vi "OCR_Find Text Row Locations.vi"(8 "Error":errorcluster, 9 "Color Array":T1[](array[typedef]), 10 "Row Type Array":T3[](array[typedef]), 11 "Frame Color":u32(colorbox)) -> (0 "Error Out":errorcluster, 1 "All Good Out":bool, 2 "Body Cluster Out":T2, 3 "Color Array Out":T1[](array[typedef]), 4 "Header Out":bool)   [LabVIEW 2009]
doc: "Finds Text Row location of each text line in the icon"
uses:
  Controls/Enum/ENUM_Line Letter Type.ctl
  Controls/Cluster/Cluster_Line Location and status.ctl
  Controls/Cluster/Cluster_Text Color Set.ctl
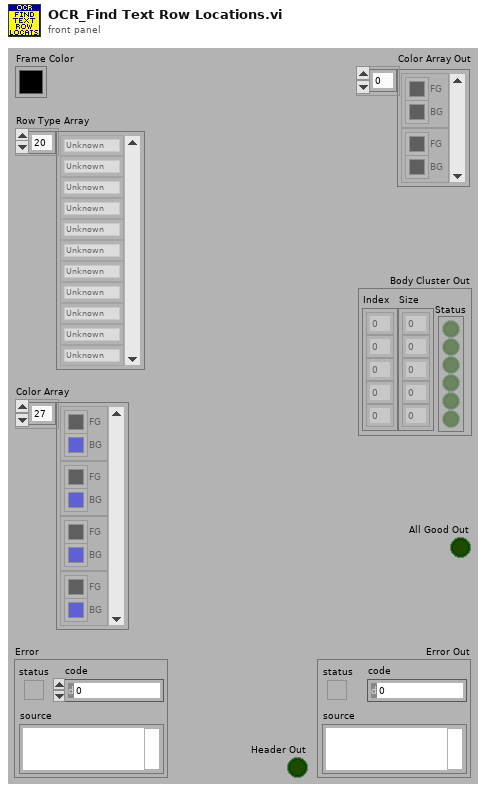
[diagram p1: front panel]
types:
  T1 = typedef "Cluster_Text Color Set.ctl" = cluster{"BG":u32, "FG":u32}
  T2 = typedef "Cluster_Line Location and status.ctl" = cluster{"Index":i16[], "Status":bool[], "Size":i32[]}
  T3 = typedef "ENUM_Line Letter Type.ctl" = enum16{"Unknown", "Letter", "Seperator", "Seperator or Letter"}
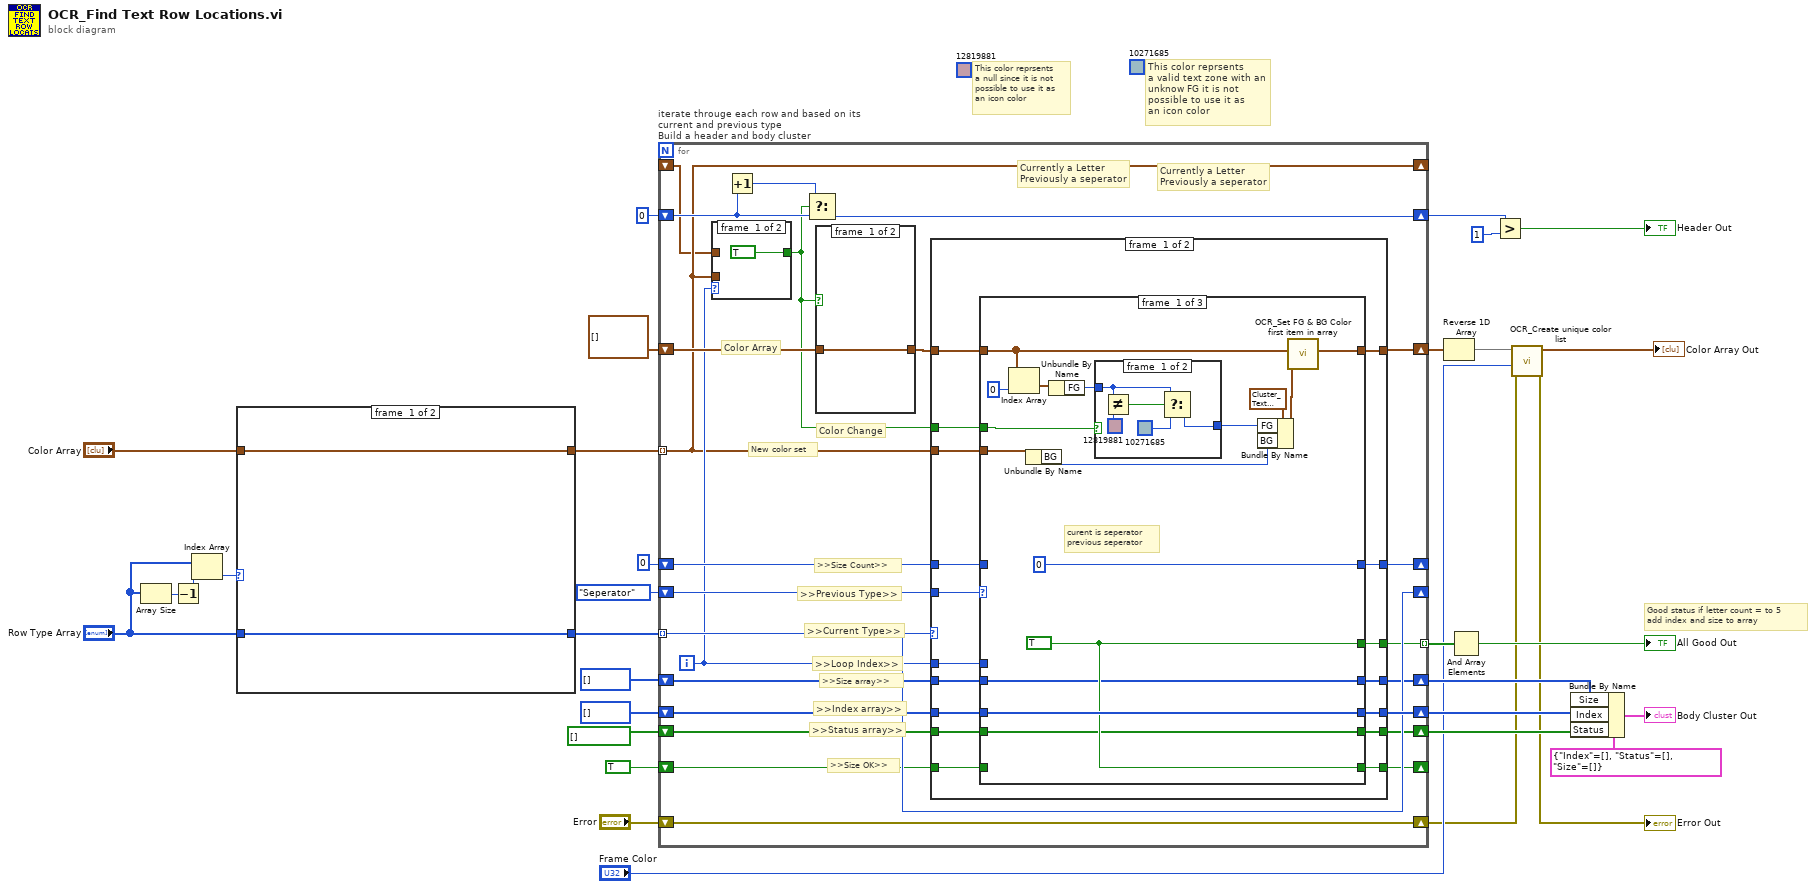
[diagram p0: block diagram]
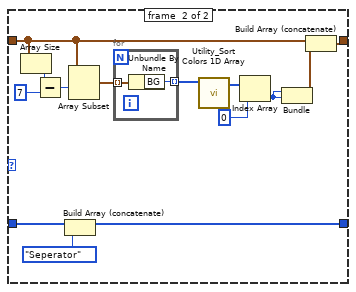
[diagram p2: hidden frame]
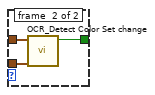
[diagram p3: hidden frame]
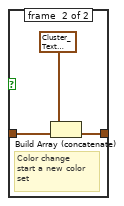
[diagram p4: hidden frame]
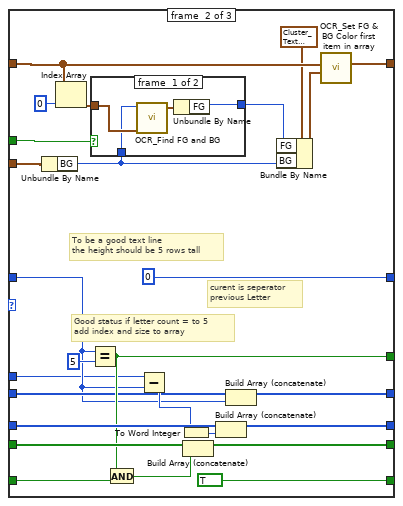
[diagram p6: hidden frame]
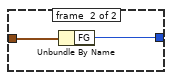
[diagram p7: hidden frame]
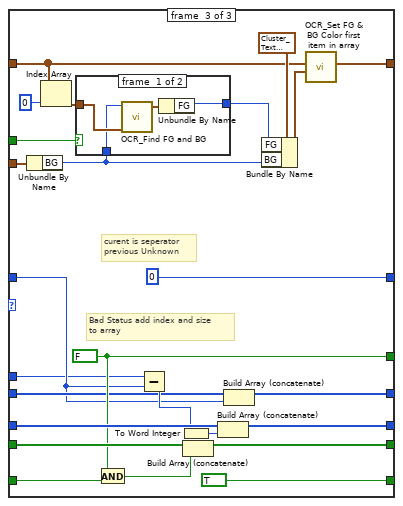
[diagram p8: hidden frame]
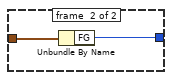
[diagram p9: hidden frame]
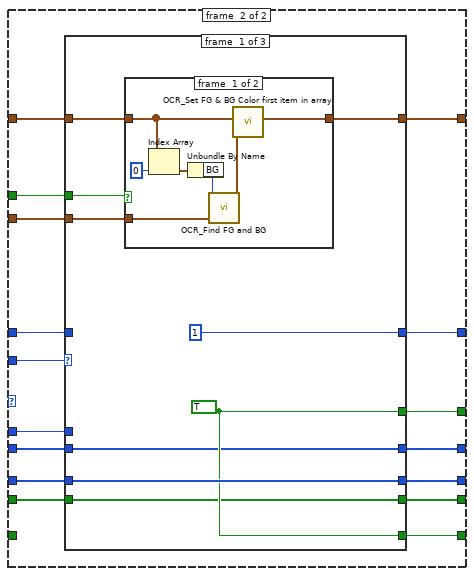
[diagram p10: hidden frame]
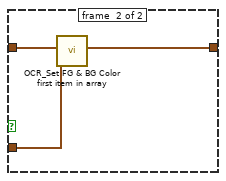
[diagram p11: hidden frame]
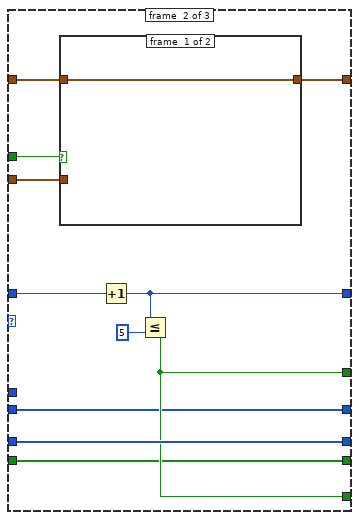
[diagram p12: hidden frame]
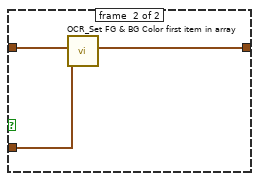
[diagram p13: hidden frame]
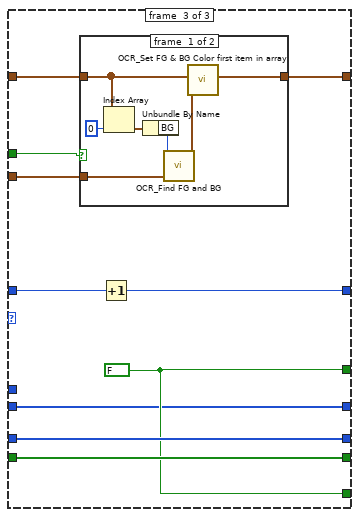
[diagram p14: hidden frame]
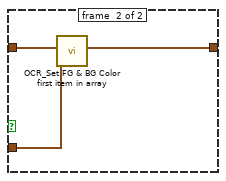
[diagram p15: hidden frame]
diagram:
  (unwired) u32 10271685 ("Unknown FG")
  (unwired) u32 12819881
  # "This color reprsents\na valid text zone with an \nunknow FG it is not\npossible to use it as\nan icon color"
  # "This color reprsents\na null since it is not\npossible to use it as\nan icon color"
  # "Good status if letter count = to 5\nadd index and size to array"
  n1 = Array Size(array="Row Type Array") -> (size(s)=w5:i32)
  n2 = Decrement(x=w5) -> (x-1=w4:i32)
  n3 = Index Array(array="Row Type Array", index=w4) -> (element=w1:T3)
  n4 = case shown="Default" w1 {
    tunnel: "Color Array" -> [w34 w44]
    tunnel: [w34 w48] -> w6
    tunnel: "Row Type Array" -> [w33 w47]
    tunnel: [w33 w46] -> w3
    frame #0 {
    }
    frame #1 {
      n5 = Array Size(array=w44) -> (size(s)=w43:i32)
      n6 = Subtract(x=w43, y=7) -> (x-y=w41:i32)
      n7 = Build Array (concatenate)(w47, ENUM_Line_Letter_Type."Seperator" ("element")) -> (w46:T3[])
      n8 = Array Subset(array=w44, index=w41) -> (w40:T1[])  [unwired: 1 in]
      n9 = for {
        tunnel: w40 -> [w50] mode=indexing
        tunnel: [w49] -> w39 mode=indexing
        n10 = Unbundle By Name(w50) -> ("BG"=w49:u32)
      }
      n11 = call "Utility_Sort Colors 1D Array.vi"("Colors"=w39) -> ("Sorted By Quantity Out"=w38:u32[])  [unwired: 8 in, 2 out]
      n12 = Index Array(array=w38, index=0) -> (element=w37:u32)
      n13 = Bundle(w37, w37) -> (w35:cluster{u32, u32})  [unwired: 1 in]
      n14 = Build Array (concatenate)(w44, w35) -> (w48:T1[])
    }
  }
  n15 = for "iterate througe each row and based on its current and previous type\nBuild a header and body cluster" {
    tunnel: w3 -> [w68] mode=indexing
    shift-right: [w74] -> w9
    shift-left: "Error" -> [w74]
    shift-right: [w71] -> _
    shift-left: 0 -> [w72]
    shift-right: [w69] -> w22
    shift-left: i16[] [] -> [w70]
    shift-right: [w68] -> _
    shift-left: ENUM_Line_Letter_Type."Seperator" ("Type Out") -> [w73]
    tunnel: [w67] -> w28 mode=indexing
    shift-right: [w65] -> w20
    shift-left: bool[] [] -> [w64]
    shift-right: [w63] -> _
    shift-left: TRUE -> [w66]
    shift-right: [w61] -> w21
    shift-left: i32[] [] -> [w62]
    tunnel: w6 -> [w52] mode=indexing
    shift-right: [w60] -> w17
    shift-left: T1[] [] -> [w55]
    shift-right: [w57] -> w15
    shift-left: 0 -> [w58]
    shift-right: [w52] -> _
    shift-left: _ -> [w51]
    i -> [w54]
    # ">>Loop Index>>"
    # "Currently a Letter\nPreviously a seperator"
    # "Currently a Letter\nPreviously a seperator"
    # "Color Change"
    # "New color set"
    # "Color Array"
    # ">>Size Count>>"
    # ">>Current Type>>"
    # ">>Previous Type>>"
    # ">>Size OK>>"
    # ">>Status array>>"
    # ">>Index array>>"
    # ">>Size array>>"
    n16 = case shown="1.." w54 {
      tunnel: [TRUE w77] -> w53
      tunnel: w52 -> [_ w78]
      tunnel: w51 -> [_ w76]
      frame #0 {
      }
      frame #1 {
        n17 = call "OCR_Detect Color Set change.vi"("New Color Set"=w78, "Previous Color Set"=w76) -> ("Color Change Out"=w77:bool)  [unwired: 9 in]
      }
    }
    n18 = Increment(x=w58) -> (x+1=w59:i32)
    n19 = Select(t=w59, s=w53, f=w58) -> (s? t:f=w57:i32)
    n20 = case shown="True" w53 {
      tunnel: w55 -> [w79 w82]
      tunnel: [w79 w81] -> w56
      frame #0 {
      }
      frame #1 {
        # "Color change\nstart a new color\nset"
        n21 = Build Array (concatenate)(T1 {"BG"=12819881, "FG"=12819881} ("Color Set"), w82) -> (w81:T1[])
      }
    }
    n22 = case shown="\"Seperator\", \"Seperator or Letter\"" w68 {
      tunnel: w73 -> [w95 w195]
      tunnel: w72 -> [w98 w199]
      tunnel: [w99 w200] -> w71
      tunnel: w54 -> [w87 w198]
      tunnel: w70 -> [w97 w197]
      tunnel: [w96 w196] -> w69
      tunnel: [w94 w194] -> w67
      tunnel: w66 -> [w93 _]
      tunnel: [w92 w192] -> w65
      tunnel: w64 -> [w91 w191]
      tunnel: [w90 w193] -> w63
      tunnel: w62 -> [w89 w190]
      tunnel: [w88 w189] -> w61
      tunnel: w56 -> [w85 w188]
      tunnel: [w83 w187] -> w60
      tunnel: w52 -> [w84 w185]
      tunnel: w53 -> [w86 w186]
      frame #0 {
        n23 = case shown="\"Letter\"" w95 {
          tunnel: [0 0 0] -> w99
          tunnel: w98 -> [_ w133 w165]
          tunnel: w87 -> [_ w132 w164]
          tunnel: w97 -> [w114 w145 w177]
          tunnel: [w114 w144 w176] -> w96
          tunnel: [w113 w137 w168] -> w94
          tunnel: w93 -> [_ w143 w175]
          tunnel: [w112 w142 w174] -> w92
          tunnel: w91 -> [w112 w141 w173]
          tunnel: [w113 TRUE TRUE] -> w90
          tunnel: [w111 w135 w166] -> w88
          tunnel: w89 -> [w111 w134 w167]
          tunnel: w86 -> [w108 w122 w156]
          tunnel: w85 -> [w105 w126 w159]
          tunnel: [w104 w125 w163] -> w83
          tunnel: w84 -> [w106 w123 w162]
          frame #0 {
            w113 = TRUE
            # "curent is seperator\nprevious seperator"
            n24 = Index Array(array=w105, index=0) -> (element=w109:T1)
            n25 = Unbundle By Name(w106) -> ("BG"=w100:u32)
            n26 = Unbundle By Name(w109) -> ("FG"=w107:u32)
            n27 = case shown="False" w108 {
              tunnel: w107 -> [w117 w121]
              tunnel: [w118 w121] -> w101
              frame #0 {
                n28 = Not Equal?(x=w117, y=u32 12819881) -> (x != y?=w119:bool)
                n29 = Select(t=w117, s=w119, f=u32 10271685) -> (s? t:f=w118:u32)
              }
              frame #1 {
              }
            }
            n30 = Bundle By Name(cluster=T1 {"BG"=12819881, "FG"=12819881} ("Color Set"), "FG"=w101, "BG"=w100) -> (w102:T1)
            n31 = call "OCR_Set FG & BG Color first item in array.vi"("Color Set"=w102, "Color Array"=w105) -> ("Color Array"=w104:T1[])  [unwired: 9 in]
          }
          frame #1 {
            # "To be a good text line\nthe height should be 5 rows tall"
            # "Good status if letter count = to 5\nadd index and size to array"
            # "curent is seperator\nprevious Letter"
            n32 = Unbundle By Name(w123) -> ("BG"=w131:u32)
            n33 = Index Array(array=w126, index=0) -> (element=w129:T1)
            n34 = Equal?(x=w133, y=5 ("x")) -> (x = y?=w137:bool)
            n35 = case shown="False" w122 {
              tunnel: w129 -> [w151 w153]
              tunnel: [w148 w152] -> w130
              tunnel: w131 -> [w150 _]
              frame #0 {
                n36 = call "OCR_Find FG and BG.vi"("Letter Color Array"=w151, "Current BG Color"=w150) -> ("Color Set"=w149:T1)  [unwired: 9 in]
                n37 = Unbundle By Name(w149) -> ("FG"=w148:u32)
              }
              frame #1 {
                n38 = Unbundle By Name(w153) -> ("FG"=w152:u32)
              }
            }
            n39 = And(x=w137, y=w143) -> (x .and. y?=w138:bool)
            n40 = Subtract(x=w132, y=w133) -> (x-y=w140:i32)
            n41 = To Word Integer(number=w140) -> (16bit integer=w139:i16)
            n42 = Build Array (concatenate)(w141, w138) -> (w142:bool[])
            n43 = Build Array (concatenate)(w145, w139) -> (w144:i16[])
            n44 = Build Array (concatenate)(w134, w133) -> (w135:i32[])
            n45 = Bundle By Name(cluster=T1 {"BG"=12819881, "FG"=12819881} ("Color Set"), "FG"=w130, "BG"=w131) -> (w127:T1)
            n46 = call "OCR_Set FG & BG Color first item in array.vi"("Color Set"=w127, "Color Array"=w126) -> ("Color Array"=w125:T1[])  [unwired: 9 in]
          }
          frame #2 {
            w168 = FALSE
            # "Bad Status add index and size\nto array"
            # "curent is seperator\nprevious Unknown"
            n47 = Unbundle By Name(w162) -> ("BG"=w154:u32)
            n48 = Index Array(array=w159, index=0) -> (element=w157:T1)
            n49 = case shown="False" w156 {
              tunnel: w157 -> [w182 w184]
              tunnel: [w179 w183] -> w155
              tunnel: w154 -> [w181 _]
              frame #0 {
                n50 = call "OCR_Find FG and BG.vi"("Letter Color Array"=w182, "Current BG Color"=w181) -> ("Color Set"=w180:T1)  [unwired: 9 in]
                n51 = Unbundle By Name(w180) -> ("FG"=w179:u32)
              }
              frame #1 {
                n52 = Unbundle By Name(w184) -> ("FG"=w183:u32)
              }
            }
            n53 = And(x=w168, y=w175) -> (x .and. y?=w170:bool)
            n54 = Subtract(x=w164, y=w165) -> (x-y=w172:i32)
            n55 = To Word Integer(number=w172) -> (16bit integer=w171:i16)
            n56 = Build Array (concatenate)(w173, w170) -> (w174:bool[])
            n57 = Build Array (concatenate)(w177, w171) -> (w176:i16[])
            n58 = Build Array (concatenate)(w167, w165) -> (w166:i32[])
            n59 = Bundle By Name(cluster=T1 {"BG"=12819881, "FG"=12819881} ("Color Set"), "FG"=w155, "BG"=w154) -> (w160:T1)
            n60 = call "OCR_Set FG & BG Color first item in array.vi"("Color Set"=w160, "Color Array"=w159) -> ("Color Array"=w163:T1[])  [unwired: 9 in]
          }
        }
      }
      frame #1 {
        n61 = case shown="\"Letter\"" w195 {
          tunnel: [1 w228 w242] -> w200
          tunnel: w199 -> [_ w230 w244]
          tunnel: w198 -> [_ _ _]
          tunnel: w197 -> [w208 w229 w243]
          tunnel: [w208 w229 w243] -> w196
          tunnel: [w207 w226 w240] -> w194
          tunnel: [w207 w226 w240] -> w193
          tunnel: [w206 w225 w241] -> w192
          tunnel: w191 -> [w206 w225 w241]
          tunnel: w190 -> [w205 w224 w239]
          tunnel: [w205 w224 w239] -> w189
          tunnel: w188 -> [w202 w222 w238]
          tunnel: [w201 w221 w237] -> w187
          tunnel: w186 -> [w204 w223 w235]
          tunnel: w185 -> [w203 w220 w236]
          frame #0 {
            w207 = TRUE
            n62 = case shown="True" w204 {
              tunnel: w203 -> [w216 w217]
              tunnel: w202 -> [w212 w219]
              tunnel: [w211 w218] -> w201
              frame #0 {
                n63 = Index Array(array=w212, index=0) -> (element=w214:T1)
                n64 = Unbundle By Name(w214) -> ("BG"=w213:u32)
                n65 = call "OCR_Find FG and BG.vi"("Letter Color Array"=w216, "Current BG Color"=w213) -> ("Color Set"=w210:T1)  [unwired: 9 in]
                n66 = call "OCR_Set FG & BG Color first item in array.vi"("Color Set"=w210, "Color Array"=w212) -> ("Color Array"=w211:T1[])  [unwired: 9 in]
              }
              frame #1 {
                n67 = call "OCR_Set FG & BG Color first item in array.vi"("Color Set"=w217, "Color Array"=w219) -> ("Color Array"=w218:T1[])  [unwired: 9 in]
              }
            }
          }
          frame #1 {
            n68 = case shown="False" w223 {
              tunnel: w222 -> [w231 w234]
              tunnel: [w231 w233] -> w221
              tunnel: w220 -> [_ w232]
              frame #0 {
              }
              frame #1 {
                n69 = call "OCR_Set FG & BG Color first item in array.vi"("Color Set"=w232, "Color Array"=w234) -> ("Color Array"=w233:T1[])  [unwired: 9 in]
              }
            }
            n70 = Increment(x=w230) -> (x+1=w228:i32)
            n71 = Less Or Equal?(x=w228, y=5) -> (x <= y?=w226:bool)
          }
          frame #2 {
            w240 = FALSE
            n72 = case shown="False" w235 {
              tunnel: w236 -> [w251 w252]
              tunnel: w238 -> [w247 w254]
              tunnel: [w246 w253] -> w237
              frame #0 {
                n73 = Index Array(array=w247, index=0) -> (element=w249:T1)
                n74 = Unbundle By Name(w249) -> ("BG"=w248:u32)
                n75 = call "OCR_Find FG and BG.vi"("Letter Color Array"=w251, "Current BG Color"=w248) -> ("Color Set"=w245:T1)  [unwired: 9 in]
                n76 = call "OCR_Set FG & BG Color first item in array.vi"("Color Set"=w245, "Color Array"=w247) -> ("Color Array"=w246:T1[])  [unwired: 9 in]
              }
              frame #1 {
                n77 = call "OCR_Set FG & BG Color first item in array.vi"("Color Set"=w252, "Color Array"=w254) -> ("Color Array"=w253:T1[])  [unwired: 9 in]
              }
            }
            n78 = Increment(x=w244) -> (x+1=w242:i32)
          }
        }
      }
    }
  }
  n79 = Reverse 1D Array(array=w17) -> (reversed array=w11:T1[])
  n80 = And Array Elements(Boolean array=w28) -> (logical AND=→"All Good Out":bool)
  n81 = Greater?(x=w15, y=1) -> (0:→"Header Out":bool)
  n82 = call "OCR_Create unique color list.vi"("Error"=w9, "Frame Color"="Frame Color", "Array"=w11) -> ("Error Out"=→"Error Out":errorcluster, "Duplicats Removed Out"=→"Color Array Out":T1[])  [unwired: 7 in]
  n83 = Bundle By Name(cluster=T2 {"Index"=[], "Status"=[], "Size"=[]} ("Location And Status Out"), "Size"=w21, "Index"=w22, "Status"=w20) -> (→"Body Cluster Out":T2)
